vi "Get Refnum From Indexing Terminal.vi"(8 "error in":errorcluster, 11 "Refnum Terminal":refnum<vi>) -> (0 "error out":errorcluster, 2 "Chosen Terminal":refnum<vi>, 3 "Terminal Data Cluster":T1)   [LabVIEW 2023]
doc: "Determine if terminal is on an indexing tunnel, and report which side of the tunnel is the refnum side (choice 1 = ouside structure, chce 2 = inside structure)\n\nThis VI returns the refnum terminal side of an indexing terminal (or the input value if it was already a refnum terminal)."
panel:
  # "non-array terminal is input is indexing"
  # "can be refnum or cluster type"
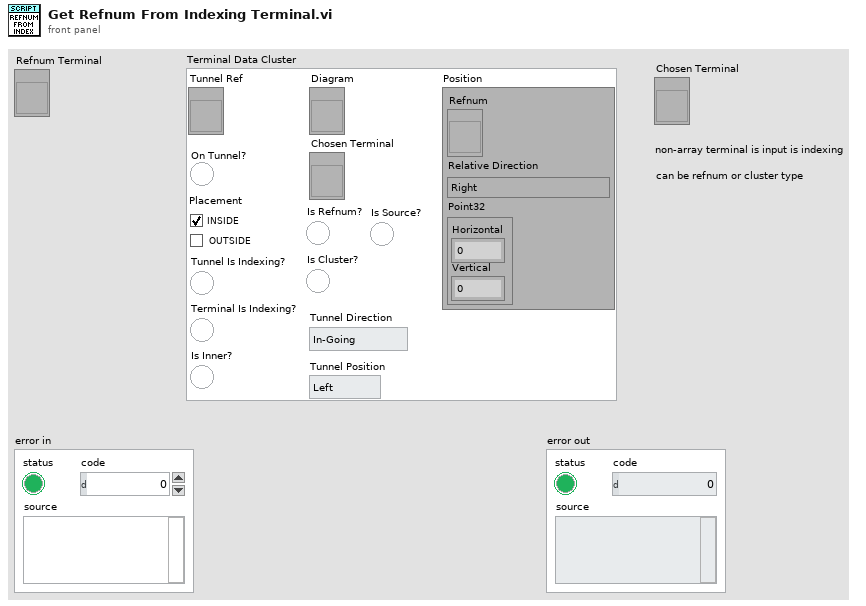
[diagram p1: front panel]
types:
  T1 = cluster{"Tunnel Ref":refnum<vi>, "On Tunnel?":bool, "Placement":enum32{"Choice 1", "Choice 2"}, "Tunnel Is Indexing?":bool, "Diagram":refnum<vi>, "Position":cluster{"Refnum":refnum<vi>, "Relative Direction":enum32{"Right", "Left", "Top", "Bottom", "Top Right", "Top Left", "Bottom Right", "Bottom Left"}, "Point32":cluster{"Horizontal":i32, "Vertical":i32}}, "Chosen Terminal":refnum<vi>, "Is Refnum?":bool, "Is Cluster?":bool, "Is Source?":bool, "Tunnel Direction":enum16{"In-Going", "Out-Going"}, "Tunnel Position":enum16{"Left", "Top", "Right", "Bottom"}, "Is Inner?":bool, "Terminal Is Indexing?":bool}
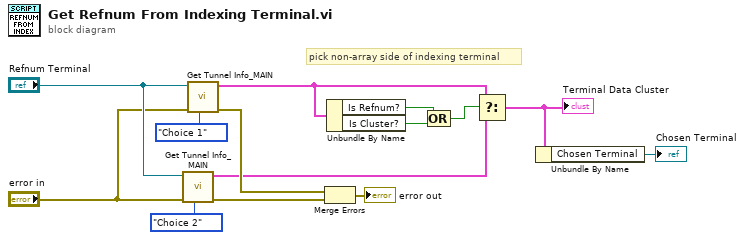
[diagram p0: block diagram]
diagram:
  # "pick non-array side of indexing terminal"
  n1 = call "Get Tunnel Info_MAIN.vi"("Object Placement"=enum32{"Choice 1", "Choice 2"}."Choice 2", "error in"="error in", "Terminal in"="Refnum Terminal") -> ("error out"=w11:errorcluster, "Terminal Data Cluster"=w8:T1)  [unwired: 6 in, 1 out]
  n2 = call "Get Tunnel Info_MAIN.vi"("Object Placement"=enum32{"Choice 1", "Choice 2"}."Choice 1", "error in"="error in", "Terminal in"="Refnum Terminal") -> ("error out"=w10:errorcluster, "Terminal Data Cluster"=w12:T1)  [unwired: 6 in, 1 out]
  n3 = Merge Errors(w10, w11) -> (→"error out":errorcluster)
  n4 = Unbundle By Name(w12) -> ("Is Refnum?"=w4:bool, "Is Cluster?"=w5:bool)
  n5 = Compound Arithmetic op=OR(w4, w5) -> (w3:bool)
  n6 = Select(t=w12, s=w3, f=w8) -> (s? t:f=w2:T1)
  "Terminal Data Cluster" <- w2
  n7 = Unbundle By Name(w2) -> ("Chosen Terminal"=→"Chosen Terminal":refnum<vi>)
